vi "软件框架.vi"() -> ()   [LabVIEW 2018]
uses:
  <vilib>/userdefined/High Color/IMAQdx.ctl
panel:
  in  "Session In":T1
  out "Image":T2(plugin-control)
  in  "安全退出":bool
  in  "采集图像":bool
  in  "打开摄像头":bool
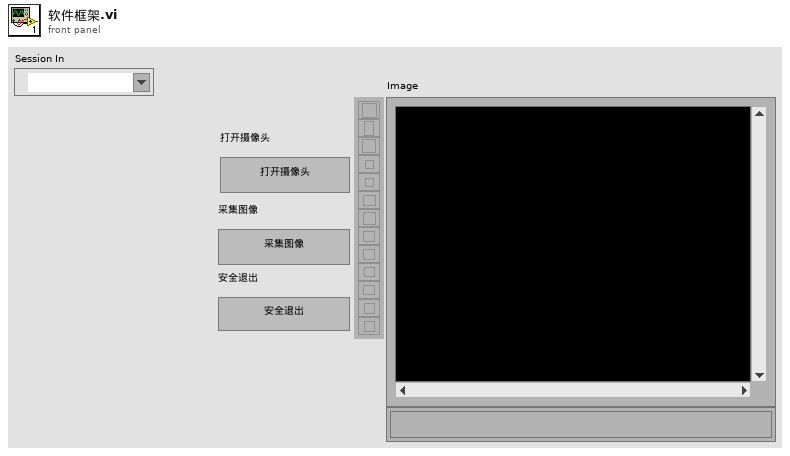
[diagram p1: front panel]
types:
  T1 = typedef "IMAQdx.ctl" = refnum<k21>
  T2 = typedef "IMAQ Image.ctl" = refnum<image>
  T3 = cluster{"queue out":refnum<queue>, "Session In":refnum<vi>, "New Image":T2}
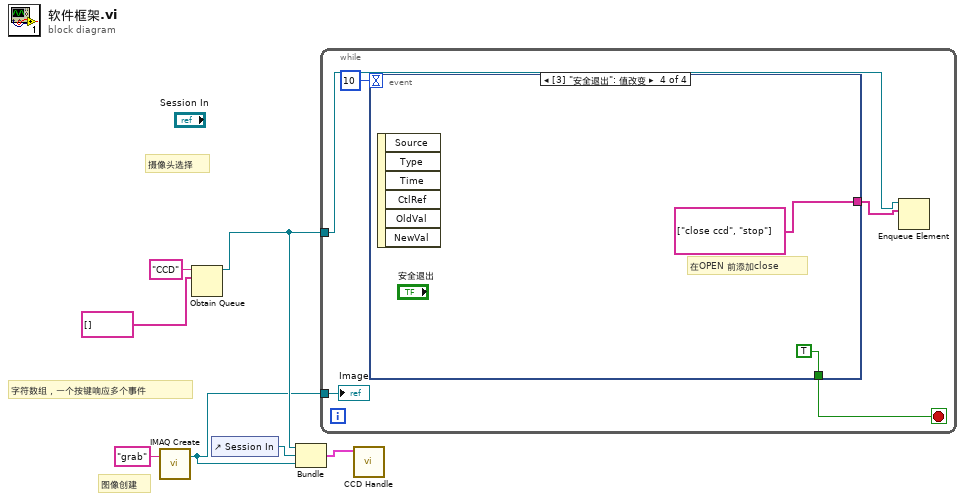
[diagram p0: block diagram]
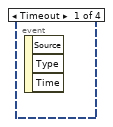
[diagram p2: hidden frame]
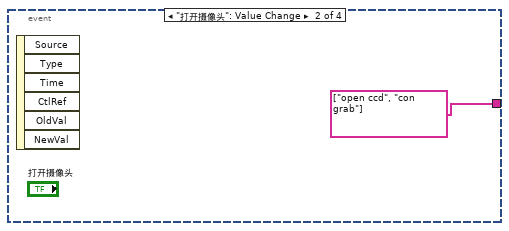
[diagram p3: hidden frame]
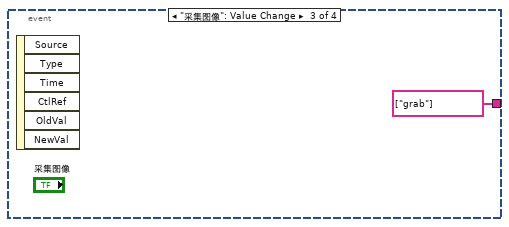
[diagram p4: hidden frame]
diagram:
  # "图像创建"
  # "摄像头选择"
  # "字符数组，一个按键响应多个事件"
  n1 = call "IMAQ Create"("Image Name"="grab") -> ("New Image"=w1:T2)  [unwired: 4 in, 1 out]
  n2 = Obtain Queue(name (unnamed)="CCD" ("名称（未命名）"), element data type=string[] []) -> (queue out=w4:refnum<queue>)  [unwired: 3 in, 2 out]
  n3 = control-ref of="Session In"() -> (w3:refnum<vi>)
  n4 = Bundle("queue out"=w4, "Session In"=w3, "New Image"=w1) -> (w2:T3)  [unwired: 1 in]
  n5 = while {
    tunnel: w4 -> [w11]
    tunnel: w1 -> [w8]
    stop <- w9 stop-if-true
    n6 = event shown="[3] \"安全退出\": 值改变" {
      selector: _ -> [_ _ _ _]
      dyn-events: _ -> [_ _ _ _]
      timeout: 10 -> [_ _ _ _]
      tunnel: [_ string[] ["open ccd", "con grab"] string[] ["grab"] string[] ["close ccd", "stop"]] -> w10
      tunnel: [_ _ _ TRUE] -> w9
      event Timeout {
        n7 = event-data() -> ()  [unwired: 1 in, 3 out]
      }
      event "打开摄像头": Value Change {
        n8 = event-data() -> ()  [unwired: 1 in, 6 out]
      }
      event "采集图像": Value Change {
        n9 = event-data() -> ()  [unwired: 1 in, 6 out]
      }
      event "安全退出": Value Change {
        # "在OPEN 前添加close"
        n10 = event-data() -> ()  [unwired: 1 in, 6 out]
      }
    }
    n11 = Enqueue Element(queue=w11, element=w10) -> ()  [unwired: 2 in, 3 out]
    "Image" <- w8
  }
  n12 = call "CCD Handle.vi"("簇"=w2) -> ()  [unwired: 11 in]
